vi "LimitLUTMax.vi"(11 "Manual LUT":cluster{u16, u16}) -> (3 "Cluster":cluster{u16, u16})   [LabVIEW 2023, in "Camera_Controller.lvlib"]
uses:
  Camera_Controller.lvclass/Camera_Controller.ctl
  Camera_Controller.lvlib
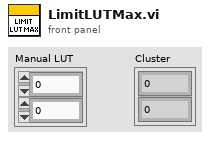
[diagram p1: front panel]
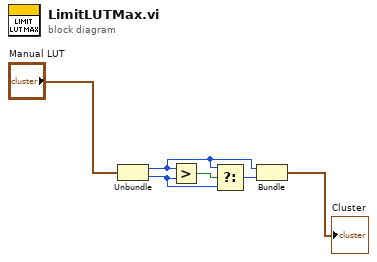
[diagram p0: block diagram]
diagram:
  n1 = Unbundle("Manual LUT") -> (w3:u16, w4:u16)
  n2 = Greater?(x=w3, y=w4) -> (0:w1:bool)
  n3 = Select(t=w3, s=w1, f=w4) -> (s? t:f=w2:u16)
  n4 = Bundle(w3, w2) -> (→"Cluster":cluster{u16, u16})  [unwired: 1 in]
